vi "AM Convert All Data From FGV.vi"(10 "Spec Temperature":dbl, 11 "Visible Plot":bool[][](array[boolean])) -> (1 "Max Temp Index":i32, 2 "SG at SPEC Temp":dbl[](array[numeric]), 3 "All Data Cluster":cluster{"Splitted Data":dbl[], dbl[]}[](array[cluster]), 4 "XY Graph":cluster{"X":dbl[], "Y":dbl[]}[][](array[cluster]), 5 "Temp Length":i32[](array[numeric]))   [LabVIEW 2020, in "Test Driver.lvlib"]
uses:
  Test Driver.lvlib
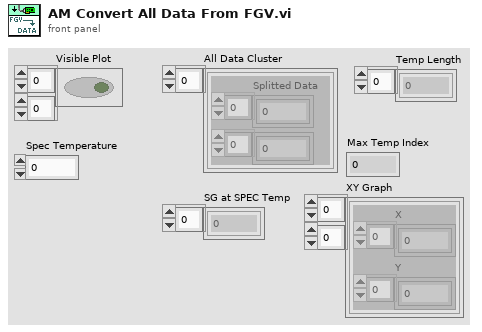
[diagram p1: front panel]
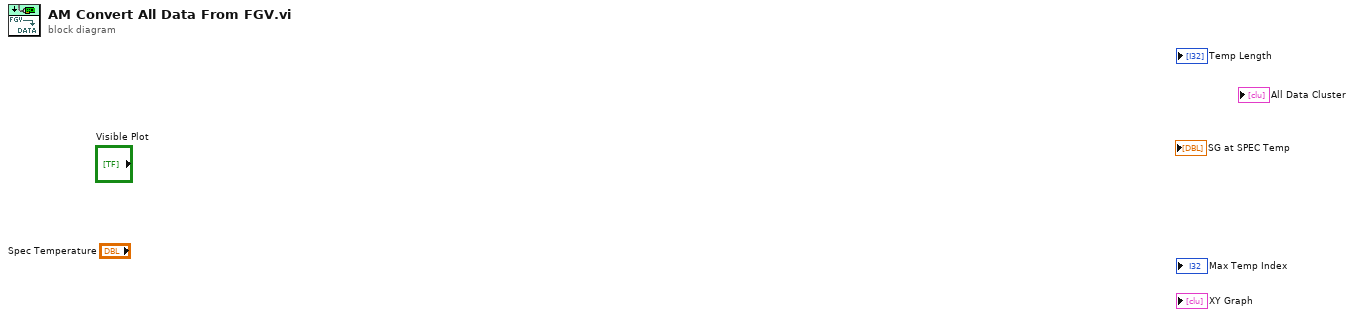
[diagram p0: block diagram]
diagram:
